vi "Point2Rect.vi"(1 "point b":cluster{"x":dbl, "y":dbl} {"y" format="%.2f"; "x" format="%.2f"}, 2 "point a":cluster{"x":dbl, "y":dbl} {"y" format="%.2f"; "x" format="%.2f"}) -> (0 "rect":T1)   [LabVIEW 2011]
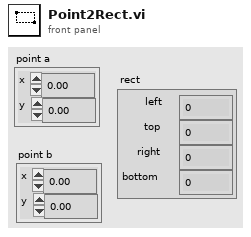
[diagram p1: front panel]
types:
  T1 = cluster{"left":i16, "top":i16, "right":i16, "bottom":i16}
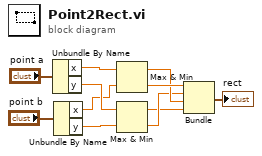
[diagram p0: block diagram]
diagram:
  n1 = Unbundle By Name("point a") -> ("x"=w8:dbl, "y"=w5:dbl)
  n2 = Unbundle By Name("point b") -> ("x"=w1:dbl, "y"=w4:dbl)
  n3 = Max & Min(x=w8, y=w1) -> (max(x,y)=w6:dbl, min(x,y)=w7:dbl)
  n4 = Max & Min(x=w5, y=w4) -> (max(x,y)=w2:dbl, min(x,y)=w3:dbl)
  n5 = Bundle(w7, w3, w6, w2) -> (→"rect":cluster{dbl, dbl, dbl, dbl})  [unwired: 1 out]
